vi "Hex to U8.vi"(1 "Hex":string) -> (0 "U8":string)   [LabVIEW 2020, in "Registration.lvclass"]
uses:
  Registration.lvclass
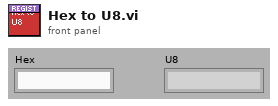
[diagram p1: front panel]
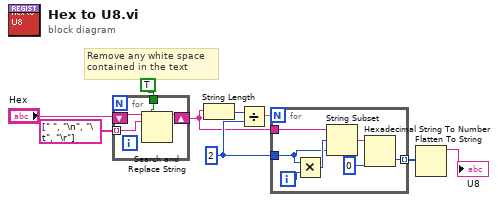
[diagram p0: block diagram]
diagram:
  w7 = 2 ("length (rest)")
  # "Remove any white space\ncontained in the text"
  n1 = for {
    tunnel: TRUE ("replace all? (F)") -> [w13]
    shift-right: [w11] -> w2
    shift-left: "Hex" -> [w12]
    tunnel: string[] [" ", "\n", "\t", "\r"] -> [w10] mode=indexing
    n2 = Search and Replace String(replace all?=w13, input string=w12, search string=w10) -> (result string=w11:string)  [unwired: 5 in, 3 out]
  }
  n3 = String Length(string=w2) -> (length=w5:i32)
  n4 = Divide(x=w5, y=w7) -> (x/y=w6:dbl)
  n5 = for {
    N: w6 -> [_]
    tunnel: w2 -> [w19]
    tunnel: [w20] -> w8 mode=indexing
    tunnel: w7 -> [w15]
    i -> [w17]
    n6 = Multiply(x=w15, y=w17) -> (x*y=w16:i32)
    n7 = String Subset(string=w19, offset (0)=w16, length (rest)=w15) -> (substring=w18:string)
    n8 = Hexadecimal String To Number(string=w18, default (0uL)=u8 0 ("default (0 U32)")) -> (number=w20:u8)  [unwired: 1 in, 1 out]
  }
  n9 = Flatten To String(anything=w8) -> (data string=→"U8":string)  [unwired: 3 in, 2 out]
